vi "Module List.vi"(8 "error in (no error)":errorcluster) -> (0 "error out":errorcluster, 3 "Modules":T1[](array[typedef]))   [LabVIEW 2018, in "Core.lvlib"]
uses:
  Core.lvlib
  Controls/Module.ctl
  Controls/Module Instance.ctl
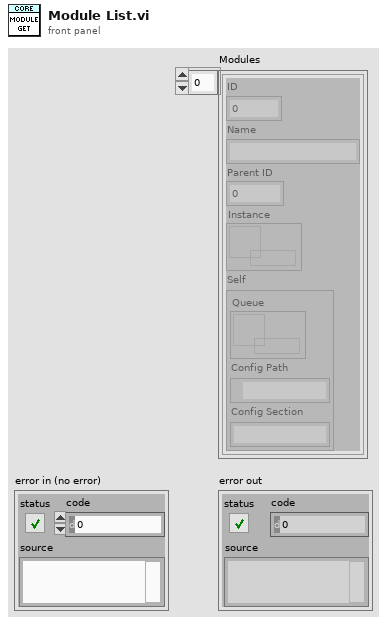
[diagram p1: front panel]
types:
  T1 = typedef "Core.lvlib/Module.ctl" = cluster{"ID":i32, "Name":string, "Parent ID":i32, "Instance":refnum<data-value>, "Self":T2}
  T2 = typedef "Core.lvlib/Module Instance.ctl" = cluster{"Queue":refnum<queue>, "Config Path":path, "Config Section":string}
  T3 = cluster{"ID":i32, "Name":string, "Parent ID":i32, "Instance":refnum<data-value>}[]
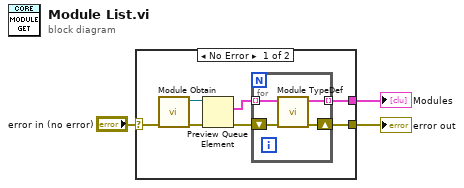
[diagram p0: block diagram]
diagram:
  n1 = case shown="No Error" "error in (no error)" {
    selector: "error in (no error)" -> [w10 w15]
    tunnel: [w7 w15] -> w2
    tunnel: [w6 _] -> w1
    frame No Error {
      n2 = call "Module Obtain.vi"("error in (no error)"=w10) -> ("error out"=w9:errorcluster, "Modules"=w8:refnum<queue>)  [unwired: 8 in, 1 out]
      n3 = Preview Queue Element(queue=w8, error in (no error)=w9) -> (element=w4:T3, error out=w5:errorcluster)  [unwired: 1 in, 2 out]
      n4 = for {
        tunnel: [w13] -> w6 mode=indexing
        shift-right: [w14] -> w7
        shift-left: w5 -> [w12]
        tunnel: w4 -> [w11] mode=indexing
        n5 = call "Module TypeDef.vi"("error in (no error)"=w12, "Module in"=w11) -> ("error out"=w14:errorcluster, "Module"=w13:T1)  [unwired: 8 in]
      }
    }
    frame Error {
    }
  }
  "error out" <- w2
  "Modules" <- w1
